vi "BubbleTeaShop_Create.vi"(8 "Error In":errorcluster, 11 "reference in":refnum<class "BubbleTeaShop.lvclass">) -> (0 "Error Out":errorcluster, 3 "reference out":refnum<class "BubbleTeaShop.lvclass">)   [LabVIEW 2020, in "BubbleTeaShop.lvclass"]
uses:
  BubbleTeaShop.lvclass
  IBeverage_interface/IBeverage.lvclass
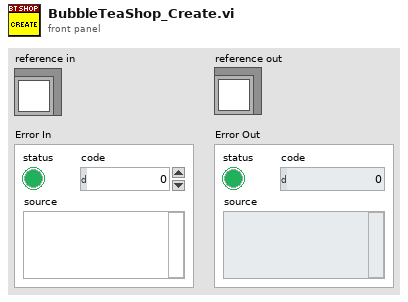
[diagram p1: front panel]
types:
  T1 = typedef "BubbleTeaShop.lvclass/ObjectAttributes.ctl" = cluster{"TakeAwayOrders":refnum<class "IBeverage.lvclass">[]}
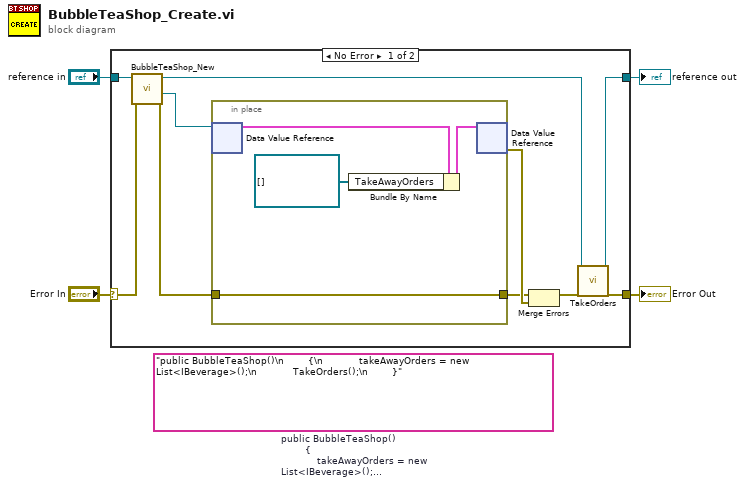
[diagram p0: block diagram]
diagram:
  (unwired) "public BubbleTeaShop()\n        {\n            takeAwayOrders = new List<IBeverage>();\n            TakeOrders();\n        }"  # public BubbleTeaShop()         {             takeAwayOrders = new List<IBeverage>();             TakeOrders();         }
  n1 = case shown="No Error" "Error In" {
    selector: "Error In" -> [w13 w20]
    tunnel: [w7 w20] -> w3
    tunnel: "reference in" -> [w14 w19]
    tunnel: [w5 w19] -> w1
    frame No Error {
      n2 = call "BubbleTeaShop_New.vi"("error in (no error)"=w13, "reference in"=w14) -> ("error out"=w10:errorcluster, "DVRRefOut"=w11:refnum<data-value>, "reference out"=w6:refnum<class "BubbleTeaShop.lvclass">)  [unwired: 6 in, 1 out]
      n3 = in-place {
        in-place-border: w10 -> [w16]
        in-place-border: [w16] -> w9
        n4 = in-place-dvr #1(w11) -> (w17:T1)  [unwired: 1 out]
        n5 = Bundle By Name(cluster=w17, "TakeAwayOrders"=refnum<class "IBeverage.lvclass">[] []) -> (w18:T1)
        n6 = in-place-dvr #1(w18) -> (w12:errorcluster)  [unwired: 1 out]
      }
      n7 = Merge Errors(w9, w12) -> (w8:errorcluster)
      n8 = call "TakeOrders.vi"("Error In"=w8, "reference in"=w6) -> ("Error Out"=w7:errorcluster, "reference out"=w5:refnum<class "BubbleTeaShop.lvclass">)  [unwired: 8 in]
    }
    frame Error {
      # "VI-TechBaseTemplate_Simple_4x4x4"
    }
  }
  "Error Out" <- w3
  "reference out" <- w1
